vi "探头偏移修正值.vi"(7 "校准参数":u16(ring) caption="校准参数：" items=["pH", "DO", "浊度", "电导率", "叶绿素a", "藻密度", "ORP", "DO2", "氯化物"], 8 "error in (no error)":errorcluster caption="错误输入（无错误）", 11 "温度偏移修正值":sgl) -> (0 "error out":errorcluster caption="错误输出")   [LabVIEW 2016, in "斯坦道多参数.lvlib"]
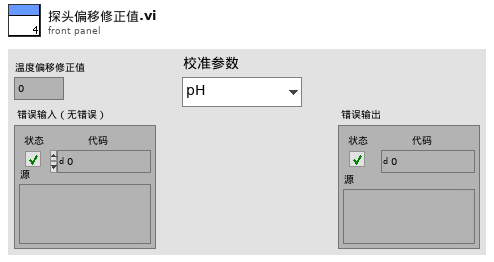
[diagram p1: front panel]
types:
  T1 = typedef "斯坦道多参数.lvlib/探头类型.ctl" = enum16{"禹山", "国弘", "纳清", "STD"}
  T2 = enum16{"NULL", "pH", "Cond", "DO", "Turb", "ORP"}
  T3 = enum16{"NULL", "pH", "Cond", "DO", "Turb", "ORP", "6", "7", "8", "9", "氯化物"}
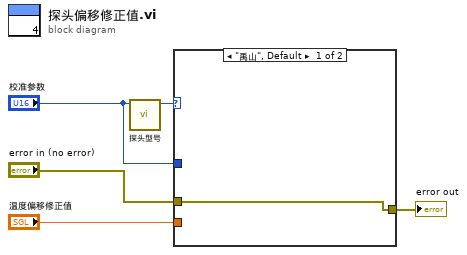
[diagram p0: block diagram]
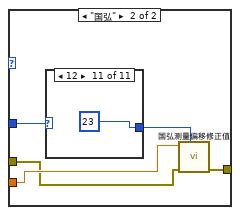
[diagram p2: hidden frame]
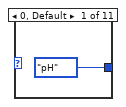
[diagram p3: hidden frame]
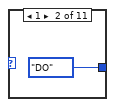
[diagram p4: hidden frame]
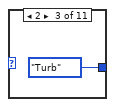
[diagram p5: hidden frame]
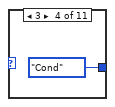
[diagram p6: hidden frame]
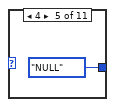
[diagram p7: hidden frame]
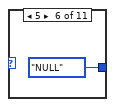
[diagram p8: hidden frame]
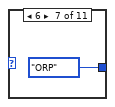
[diagram p9: hidden frame]
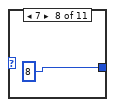
[diagram p10: hidden frame]
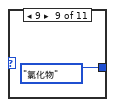
[diagram p11: hidden frame]
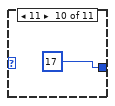
[diagram p12: hidden frame]
diagram:
  n1 = call "探头型号.vi"("校准参数"="校准参数") -> ("探头型号"=w5:T1)  [unwired: 8 in, 2 out]
  n2 = case shown="\"禹山\", Default" w5 {
    tunnel: "校准参数" -> [_ w11]
    tunnel: "error in (no error)" -> [w6 w7]
    tunnel: [w6 w8] -> w2
    tunnel: "温度偏移修正值" -> [_ w9]
    frame "禹山", Default {
    }
    frame "国弘" {
      n3 = case shown="12" w11 {
        tunnel: [T2."pH" ("探头") T2."DO" ("探头") T2."Turb" ("探头") T2."Cond" ("探头") T2."NULL" ("探头") T2."NULL" ("探头") T2."ORP" ("探头") 8 T3."氯化物" ("探头") 17 23] -> w10
        frame 0, Default {
        }
        frame 1 {
        }
        frame 2 {
        }
        frame 3 {
        }
        frame 4 {
        }
        frame 5 {
        }
        frame 6 {
        }
        frame 7 {
        }
        frame 9 {
        }
        frame 11 {
        }
        frame 12 {
        }
      }
      n4 = call "国弘测量偏移修正值.vi"("探头"=w10, "error in (no error)"=w7, "温度偏移修正值"=w9) -> ("error out"=w8:errorcluster)  [unwired: 7 in, 1 out]
    }
  }
  "error out" <- w2
